vi "Clean Build.vi"   [LabVIEW 2020]
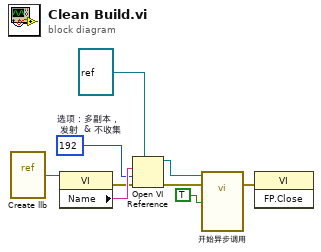
[diagram p0: block diagram]
diagram:
  w4 = 192  # 选项：多副本，  发射  & 不收集
  n1 = vi-ref "Create llb.vi"() -> (w8:refnum<vi>)
  n2 = property class="VI"(reference=w8) -> (error out=w3:errorcluster, "Name"=w9:string)  [unwired: 1 in, 1 out]
  n3 = Open VI Reference(type specifier VI Refnum (for type only)=refnum<vi> refnum ("引用"), vi path=w9, options=w4, error in (no error)=w3) -> (vi reference=w5:refnum<vi>, error out=w2:errorcluster)  [unwired: 2 in]
  n4 = call-by-ref "开始异步调用"(reference=w5, error in=w2, "Clean Build"=TRUE) -> (error out=w1:errorcluster)  [unwired: 11 in, 1 out]
  n5 = invoke class="VI" method="FP.Close"(error in=w1) -> ()  [unwired: 2 in, 3 out]
